vi "Update Window Title.vi"(8 "error in (no error)":errorcluster, 9 "Experiment Name":string, 10 "Experiment File Path":path, 11 "VI in":refnum<vi>) -> (0 "error out":errorcluster)   [LabVIEW 2020]
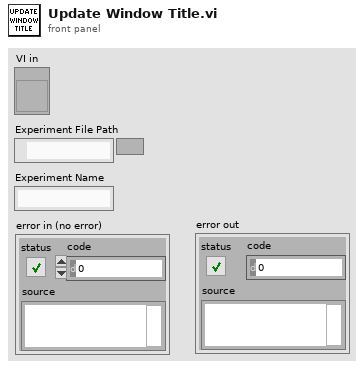
[diagram p1: front panel]
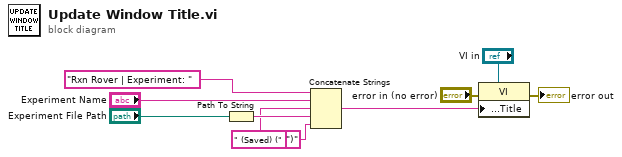
[diagram p0: block diagram]
diagram:
  n1 = Path To String(path="Experiment File Path") -> (string=w9:string)
  n2 = Concatenate Strings("Rxn Rover | Experiment: ", "Experiment Name", " (Saved) (", w9, ")") -> (w6:string)
  n3 = property class="VI"(reference="VI in", error in="error in (no error)", "Front Panel.Title"=w6) -> (error out=→"error out":errorcluster)  [unwired: 1 out]
